vi "ReadViRef.vi"(8 "error in (no error)":errorcluster caption="错误输入（无错误）", 11 "Config Worker 输入":refnum<class "Config Worker.lvclass">) -> (0 "error out":errorcluster caption="错误输出", 2 "VI":refnum<vi>, 3 "Config Worker 输出":refnum<class "Config Worker.lvclass">)   [LabVIEW 2018, in "Config Worker.lvclass"]
uses:
  Config Worker.lvclass
  Config Worker.lvclass/Config Worker.ctl
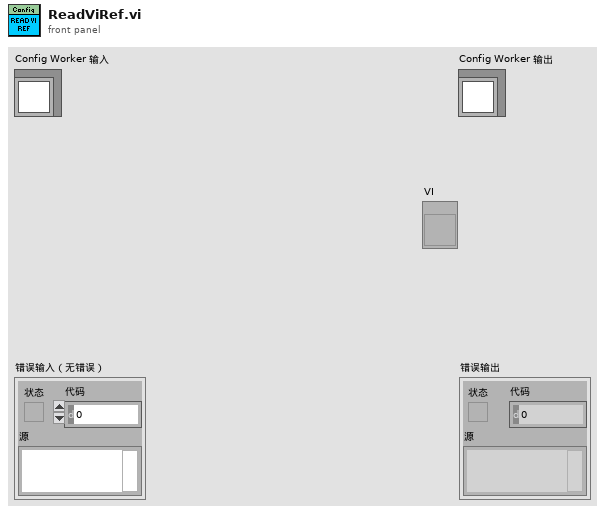
[diagram p1: front panel]
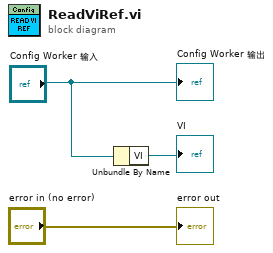
[diagram p0: block diagram]
diagram:
  n1 = Unbundle By Name("Config Worker 输入") -> ("VI"=→"VI":refnum<vi>)
  "error out" <- "error in (no error)"
  "Config Worker 输出" <- "Config Worker 输入"
